vi "Type Characters.vi"(0 "Key Array":T1(array[cluster]), 7 "Length of Key Press (ms)":u32, 11 "error in":errorcluster) -> (15 "error out":errorcluster)   [LabVIEW 2016, in "Drona.lvlib"]
doc: "Handle the actions configured in the key array control for each of the configured keys"
uses:
  Drona.lvlib
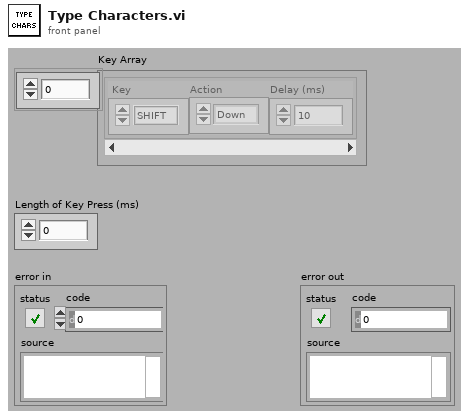
[diagram p1: front panel]
types:
  T1 = cluster{" Key":u8, "Action":enum16{"Press", "Up", "Down"}, "Delay (ms)":u32}[]
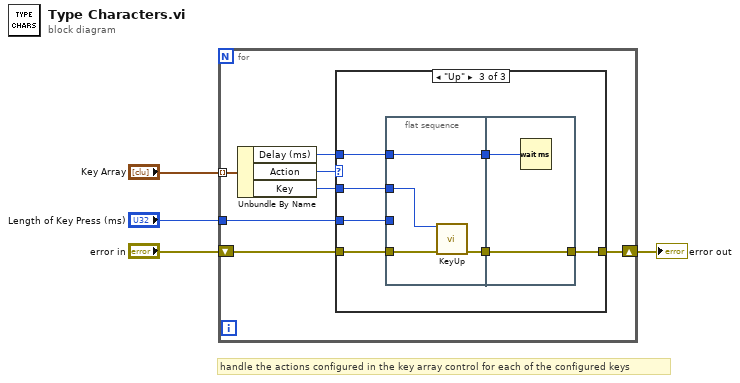
[diagram p0: block diagram]
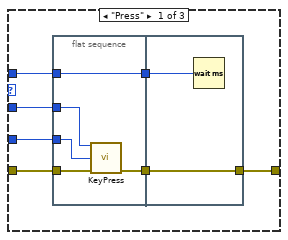
[diagram p2: hidden frame]
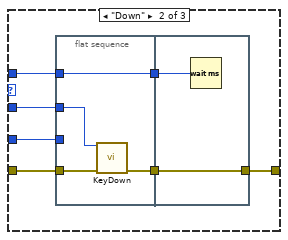
[diagram p3: hidden frame]
diagram:
  # "handle the actions configured in the key array control for each of the configured keys"
  n1 = for {
    tunnel: "Key Array" -> [w11] mode=indexing
    tunnel: "Length of Key Press (ms)" -> [w10]
    shift-right: [w5] -> w1
    shift-left: "error in" -> [w6]
    n2 = Unbundle By Name(w11) -> ("Delay (ms)"=w7:u32, "Action"=w9:enum16{"Press", "Up", "Down"}, "Key"=w8:u8)
    n3 = case shown="\"Up\"" w9 {
      tunnel: w10 -> [w18 w32 w45]
      tunnel: w8 -> [w17 w31 w44]
      tunnel: w7 -> [w15 w29 w42]
      tunnel: w6 -> [w13 w27 w41]
      tunnel: [w12 w26 w39] -> w5
      frame "Press" {
        n4 = flat-sequence {
          tunnel: w18 -> [w20]
          tunnel: w17 -> [w19]
          tunnel: [w23] -> w16
          tunnel: w15 -> [w23]
          tunnel: [w21] -> w14
          tunnel: w13 -> [w22]
          tunnel: w16 -> [w25]
          tunnel: w14 -> [w24]
          tunnel: [w24] -> w12
          frame #0 {
            n5 = call "KeyPress.vi"("Virtual Key"=w19, "Millis"=w20, "error in"=w22) -> ("error out"=w21:errorcluster)  [unwired: 12 in]
          }
          frame #1 {
            n6 = Wait (ms)(milliseconds to wait=w25) -> ()  [unwired: 1 out]
          }
        }
      }
      frame "Down" {
        n7 = flat-sequence {
          tunnel: w32 -> [_]
          tunnel: w31 -> [w35]
          tunnel: [w36] -> w30
          tunnel: w29 -> [w36]
          tunnel: [w33] -> w28
          tunnel: w27 -> [w34]
          tunnel: w30 -> [w38]
          tunnel: w28 -> [w37]
          tunnel: [w37] -> w26
          frame #0 {
            n8 = call "KeyDown.vi"("Virtual Key"=w35, "error in"=w34) -> ("error out"=w33:errorcluster)  [unwired: 13 in]
          }
          frame #1 {
            n9 = Wait (ms)(milliseconds to wait=w38) -> ()  [unwired: 1 out]
          }
        }
      }
      frame "Up" {
        n10 = flat-sequence {
          tunnel: w45 -> [_]
          tunnel: w44 -> [w48]
          tunnel: [w49] -> w43
          tunnel: w42 -> [w49]
          tunnel: w41 -> [w47]
          tunnel: [w46] -> w40
          tunnel: w43 -> [w51]
          tunnel: w40 -> [w50]
          tunnel: [w50] -> w39
          frame #0 {
            n11 = call "KeyUp.vi"("Virtual Key"=w48, "error in"=w47) -> ("error out"=w46:errorcluster)  [unwired: 13 in]
          }
          frame #1 {
            n12 = Wait (ms)(milliseconds to wait=w51) -> ()  [unwired: 1 out]
          }
        }
      }
    }
  }
  "error out" <- w1
